vi "xy_raster_scan_dynamic_retract.vi"(4 "RetractMap um":dbl[][](array[numeric]), 6 "YOffset um":dbl format="%#_13g", 7 "XOffset um":dbl format="%#_13g", 8 "YStepSize um":dbl format="%#_13g", 9 "XStepSize um":dbl format="%#_13g", 10 "YNum":i32, 11 "XNum":i32) -> (3 "Converted_HTT_Params":fxp<+/-,48,16>[](array[numeric]))   [LabVIEW 2024]
panel:
  out "appended array":dbl[][](array[numeric])
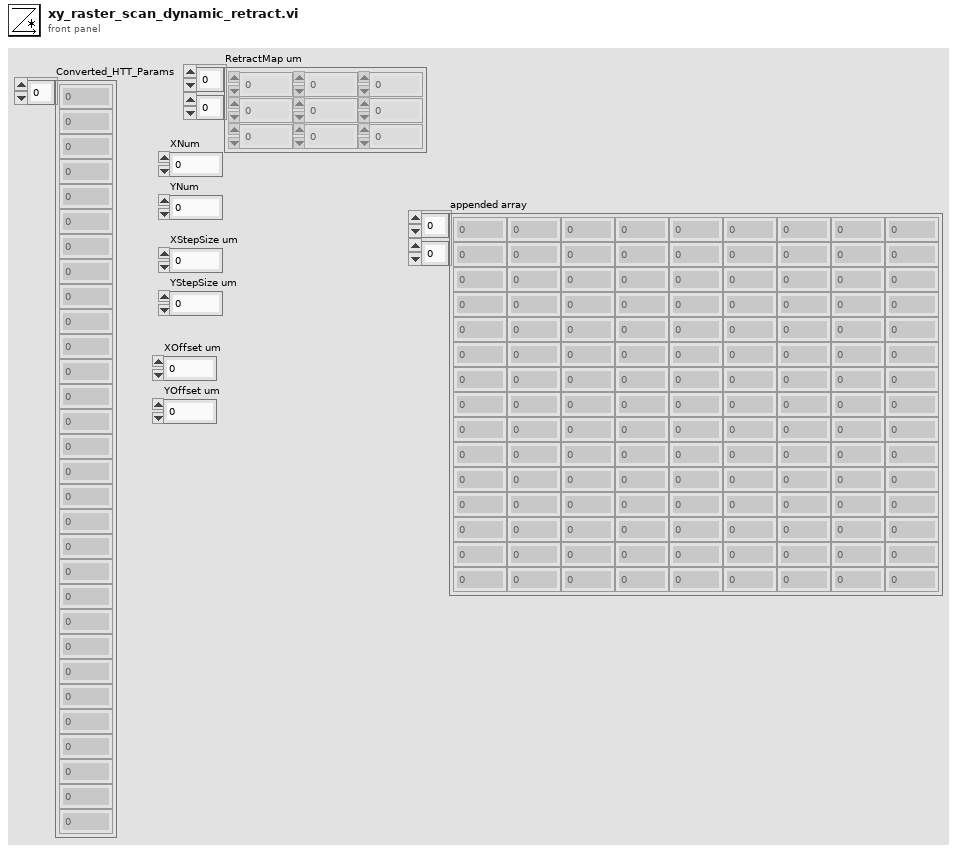
[diagram p1: front panel]
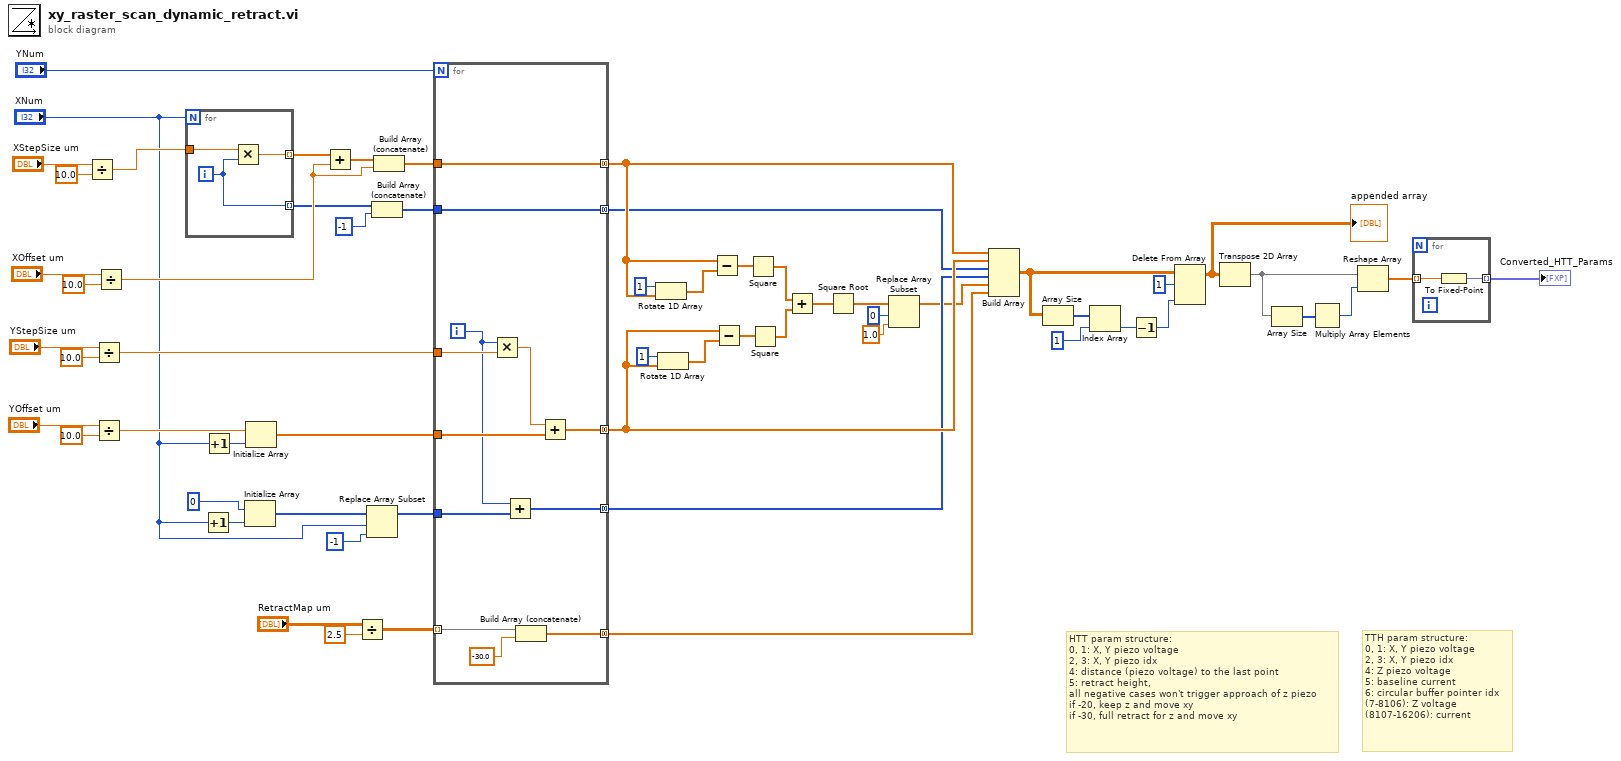
[diagram p0: block diagram]
diagram:
  # "TTH param structure:\n0, 1: X, Y piezo voltage\n2, 3: X, Y piezo idx\n4: Z piezo voltage\n5: baseline current\n6: circular buffer pointer idx\n(7-8106): Z voltage\n(8107-16206): current"
  # "HTT param structure:\n0, 1: X, Y piezo voltage\n2, 3: X, Y piezo idx\n4: distance (piezo voltage) to the last point\n5: retract height, \nall negative cases won't trigger approach of z piezo\nif -20, keep z and move xy\nif -30, full retract for z and move xy"
  n1 = Divide(x="XStepSize um", y=10.0) -> (x/y=w50:dbl)
  n2 = Divide(x="YStepSize um", y=10.0) -> (x/y=w42:dbl)
  n3 = Divide(x="YOffset um", y=10.0) -> (x/y=w41:dbl)
  n4 = Divide(x="XOffset um", y=10.0) -> (x/y=w47:dbl)
  n5 = for {
    N: "XNum" -> [_]
    tunnel: w50 -> [w63]
    tunnel: [w62] -> w49 mode=indexing
    tunnel: [w61] -> w46 mode=indexing
    i -> [w61]
    n6 = Multiply(x=w63, y=w61) -> (x*y=w62:dbl)
  }
  n7 = Increment(x="XNum") -> (x+1=w38:i32)
  n8 = Increment(x="XNum") -> (x+1=w40:i32)
  n9 = Initialize Array(0, w38) -> (w16:i32[])
  n10 = Initialize Array(w41, w40) -> (w39:dbl[])
  n11 = Add(x=w49, y=w47) -> (x+y=w48:dbl[])
  n12 = Divide(x="RetractMap um", y=2.5) -> (x/y=w2:dbl[][])
  n13 = Replace Array Subset(array=w16, new element=-1, index="XNum") -> (w15:i32[])
  n14 = Build Array (concatenate)(w46, -1) -> (w43:i32[])
  n15 = Build Array (concatenate)(w48, w47) -> (w44:dbl[])
  n16 = for {
    N: "YNum" -> [_]
    tunnel: w44 -> [w75]
    tunnel: w43 -> [w74]
    tunnel: [w75] -> w24 mode=concatenating
    tunnel: [w74] -> w22 mode=concatenating
    tunnel: w42 -> [w73]
    tunnel: w39 -> [w72]
    tunnel: [w70] -> w23 mode=concatenating
    tunnel: w15 -> [w68]
    tunnel: [w67] -> w21 mode=concatenating
    tunnel: w2 -> [w66] mode=indexing
    tunnel: [w64] -> w1 mode=concatenating
    i -> [w69]
    n17 = Multiply(x=w69, y=w73) -> (x*y=w71:dbl)
    n18 = Add(x=w69, y=w68) -> (x+y=w67:i32[])
    n19 = Build Array (concatenate)(w66, -30.0 ("new element/subarray")) -> (w64:dbl[])
    n20 = Add(x=w71, y=w72) -> (x+y=w70:dbl[])
  }
  n21 = Rotate 1D Array(1:w24, 2:1 ("n")) -> (0:w35:dbl[])
  n22 = Rotate 1D Array(1:w23, 2:1 ("n")) -> (0:w34:dbl[])
  n23 = Subtract(x=w24, y=w35) -> (x-y=w32:dbl[])
  n24 = Subtract(x=w23, y=w34) -> (x-y=w31:dbl[])
  n25 = Square(x=w32) -> (x^2=w30:dbl[])
  n26 = Square(x=w31) -> (x^2=w29:dbl[])
  n27 = Add(x=w30, y=w29) -> (x+y=w28:dbl[])
  n28 = Square Root(x=w28) -> (sqrt(x)=w27:dbl[])
  n29 = Replace Array Subset(array=w27, new element=1.0 ("new element/subarray"), index=0) -> (w20:dbl[])
  n30 = Build Array(w24, w23, w22, w21, w20, w1) -> (w10:dbl[][])
  n31 = Array Size(array=w10) -> (size(s)=w9:i32[])
  n32 = Index Array(array=w9, index=1) -> (element=w7:i32)
  n33 = Decrement(x=w7) -> (x-1=w6:i32)
  n34 = Delete From Array(array=w10, length=1, index (col)=w6) -> (array with subset deleted=w4:dbl[][])  [unwired: 1 in, 1 out]
  "appended array" <- w4
  n35 = Transpose 2D Array(2D array=w4) -> (transposed array=w5:dbl[][])
  n36 = Array Size(array=w5) -> (size(s)=w19:i32[])
  n37 = Multiply Array Elements(1:w19) -> (0:w11:i32)
  n38 = Reshape Array(w5, w11) -> (w18:dbl[])
  n39 = for {
    tunnel: w18 -> [w77] mode=indexing
    tunnel: [w76] -> w17 mode=indexing
    n40 = To Fixed-Point(number=w77) -> (fixed-point=w76:fxp<+/-,48,16>)  [unwired: 1 in]
  }
  "Converted_HTT_Params" <- w17
